vi "ControlBoardReadWrite.vi"(8 "error in (no error)":errorcluster, 10 "PWM Outputs":u8[](array[slide]) scale=0.0..255.0, 11 "LED Outputs":bool[](array[boolean])) -> (0 "error out":errorcluster, 2 "Analog Inputs":u8[](array[slide]) scale=0.0..255.0, 3 "Switch Inputs":bool[](array[boolean]))   [LabVIEW 2017]
uses:
  <vilib>/Rock Robotics/Network Tables/NT Read Boolean Array.vi
  <vilib>/Rock Robotics/Network Tables/NT Read Numeric Array.vi
  <vilib>/Rock Robotics/Network Tables/NT Write Numeric Array.vi
  <vilib>/Rock Robotics/Network Tables/NT Write Boolean Array.vi
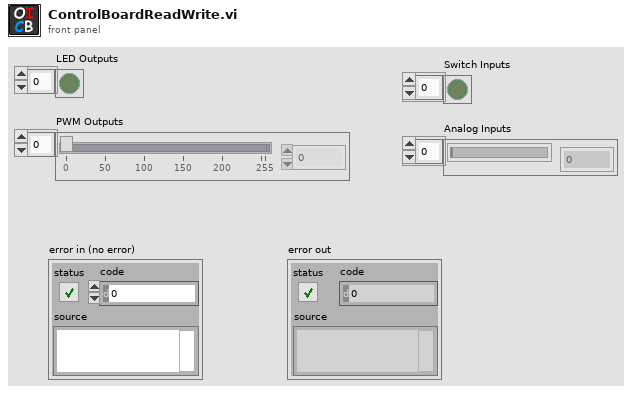
[diagram p1: front panel]
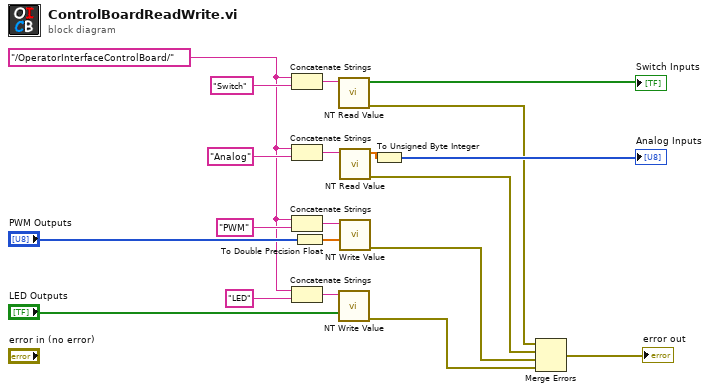
[diagram p0: block diagram]
diagram:
  w5 = "/OperatorInterfaceControlBoard/"
  n1 = Concatenate Strings(w5, "Switch" ("string")) -> (w10:string)
  n2 = Concatenate Strings(w5, "Analog" ("string")) -> (w11:string)
  n3 = Concatenate Strings(w5, "PWM" ("string")) -> (w12:string)
  n4 = Concatenate Strings(w5, "LED" ("string")) -> (w13:string)
  n5 = To Double Precision Float(number="PWM Outputs") -> (double precision float=w15:dbl[])
  n6 = call-poly <vilib>:"NT Read Value.vi"("Name"=w10) -> ("error out"=w4:errorcluster, "Boolean Array"=→"Switch Inputs":bool[])  [unwired: 9 in]
  n7 = call-poly <vilib>:"NT Write Value.vi"("Boolean Array"="LED Outputs", "Name"=w13) -> ("error out"=w1:errorcluster)  [unwired: 9 in]
  n8 = call-poly <vilib>:"NT Read Value.vi"("Name"=w11) -> ("error out"=w3:errorcluster, "Numeric Array"=w14:dbl[])  [unwired: 9 in]
  n9 = call-poly <vilib>:"NT Write Value.vi"("Numeric Array"=w15, "Name"=w12) -> ("error out"=w2:errorcluster)  [unwired: 9 in]
  n10 = To Unsigned Byte Integer(number=w14) -> (unsigned 8bit integer=→"Analog Inputs":u8[])
  n11 = Merge Errors(w4, w3, w2, w1) -> (→"error out":errorcluster)
